vi "GT Set Compare Port.vi"(7 "hsio1":i16, 8 "error in (no error)":errorcluster caption="错误输入（无错误）", 9 "hsio0":i16, 10 "channel":i16, 11 "cardNum":i16) -> (0 "error out":errorcluster caption="错误输出", 3 "function return":i16)   [LabVIEW 2014, in "gts.lvlib"]
doc: "GT_API GT_SetComparePort(short cardNum,short channel,short hsio0,short hsio1);"
uses:
  gts.lvlib
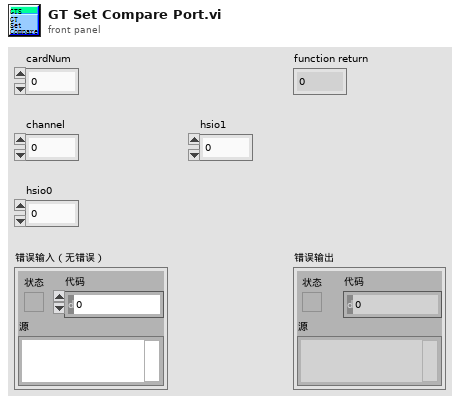
[diagram p1: front panel]
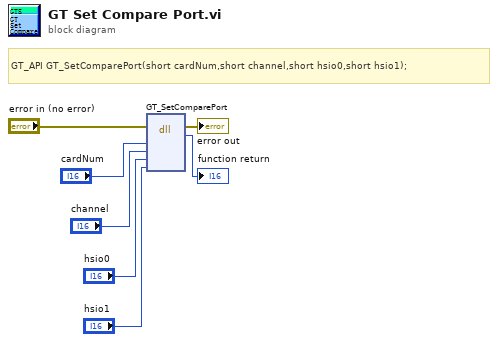
[diagram p0: block diagram]
diagram:
  # "GT_API GT_SetComparePort(short cardNum,short channel,short hsio0,short hsio1);"
  n1 = dll-call lib="PTH2habs D固高科技资料GTS控制卡GTS卡18年上半年资料dllVC32bit\nmulti_cardgts.*" fn="GT_SetComparePort"(error in="error in (no error)", "cardNum"="cardNum", "channel"="channel", "hsio0"="hsio0", "hsio1"="hsio1") -> (error out=→"error out":errorcluster, →"function return":i16)  [unwired: 6 in, 1 out]
